vi "classes.vi"(0 "HB_PollingAgent_Factory":refnum<class "HB_PollingAgent_Factory.lvclass">, 1 "className":string, 5 "error in (no error)":errorcluster) -> (14 "HB_PollingAgent_Factory dup":refnum<class "HB_PollingAgent_Factory.lvclass">, 16 "Object":refnum<class>, 19 "error out":errorcluster)   [LabVIEW 2009, in "HB_PollingAgent.lvlib" / "HB_PollingAgent_Factory.lvclass"]
doc: "This dynamaic dispatch VI contains constant objects of all classes that can be produced by HGF_Factory.\nClass has to be defined by name. \n\nOptionally, you can also specifiy a Class Path String instead, but you have to make sure that all dependencies are available.\n\nChild classes have to override it to define additional classes."
uses:
  HB_PollingAgent_Factory.lvclass
  HB_PollingAgent/HB_PollingAgent.lvclass
  HB_PollingAgentVisitor/HB_PollingAgentVisitor.lvclass
  lib.lib/HGF_LVC/HGF_MobileAgentSystem/MoAgSy_Factory/MoAgSy_Factory.lvclass
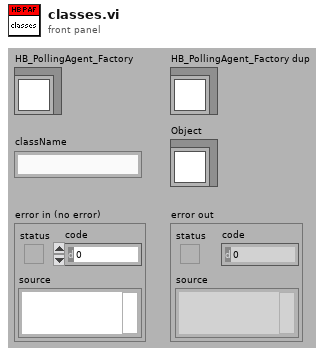
[diagram p1: front panel]
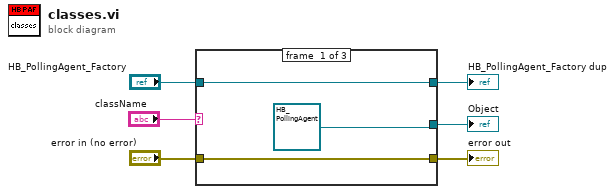
[diagram p0: block diagram]
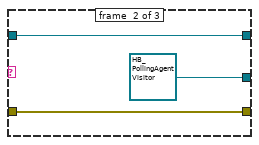
[diagram p2: hidden frame]
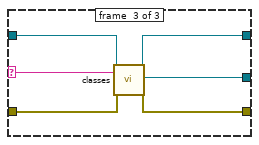
[diagram p3: hidden frame]
diagram:
  n1 = case shown="\"HB_PollingAgentVisitor\"" "className" {
    selector: "className" -> [_ _ w13]
    tunnel: "HB_PollingAgent_Factory" -> [w8 w11 w18]
    tunnel: "error in (no error)" -> [w7 w10 w17]
    tunnel: [w8 w11 w16] -> w4
    tunnel: [refnum<class "HB_PollingAgent.lvclass"> refnum ("HB_PollingAgent.lvlib:HB_PollingAgent.lvclass") refnum<class "HB_PollingAgentVisitor.lvclass"> refnum ("HB_PollingAgent.lvlib:HB_PollingAgentVisitor.lvclass") w15] -> w3
    tunnel: [w7 w10 w14] -> w2
    frame #0 {
    }
    frame #1 {
    }
    frame #2 {
      n2 = call-parent "classes.vi"("MoAgSy_Factory"=w18, "className"=w13, "error in (no error)"=w17) -> ("MoAgSy_Factory dup"=w16:refnum<class "HB_PollingAgent_Factory.lvclass">, "Object"=w15:refnum<class>, "error out"=w14:errorcluster)  [unwired: 14 in]
    }
  }
  "error out" <- w2
  "HB_PollingAgent_Factory dup" <- w4
  "Object" <- w3
